vi "SMO Base Test Launcher.vi"() -> ()   [LabVIEW 2013]
uses:
  SMO.lvclass
  Typedefs/SMOState --Enum.ctl
panel:
  out "error out":errorcluster
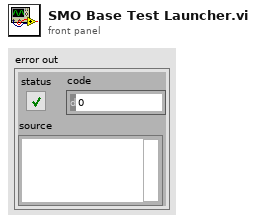
[diagram p1: front panel]
types:
  T1 = typedef "SMO.lvclass/Public Events.ctl" = cluster{"Error":refnum<user-event>, "State":refnum<user-event>, "Reserve State":refnum<user-event>}
  T2 = cluster{"Event Registration Refnum":refnum<event-registration>}
  T3 = typedef "SMO.lvclass/SMOState --Enum.ctl" = enum16{"unknown", "Created", "Started", "Stopped"}
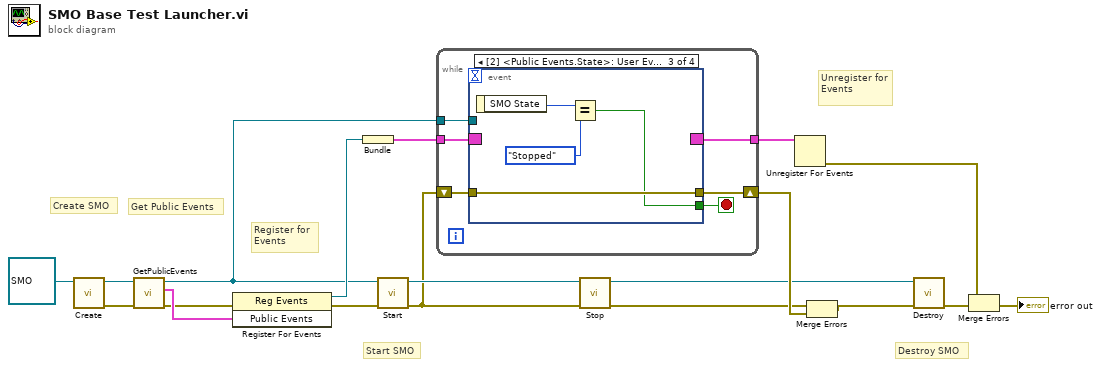
[diagram p0: block diagram]
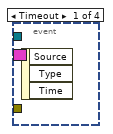
[diagram p2: hidden frame]
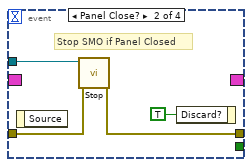
[diagram p3: hidden frame]
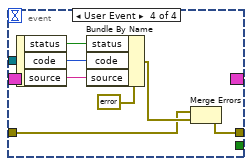
[diagram p4: hidden frame]
diagram:
  # "Get Public Events"
  # "Start SMO"
  # "Destroy SMO"
  # "Create SMO"
  # "Unregister for Events"
  # "Register for Events"
  n1 = call "Create.vi"("SMO"=refnum<class "SMO.lvclass"> refnum) -> ("error out"=w11:errorcluster, "SMO out"=w10:refnum<class "SMO.lvclass">)  [unwired: 8 in, 1 out]
  n2 = call "GetPublicEvents.vi"("error in (no error)"=w11, "SMO"=w10) -> ("error out"=w7:errorcluster, "Public Events"=w9:T1, "SMO out"=w8:refnum<class "SMO.lvclass">)  [unwired: 7 in]
  n3 = register-events(error in=w7, w9) -> (reference out=w13:refnum<event-registration>, error out=w12:errorcluster)  [unwired: 1 in]
  n4 = Bundle("Event Registration Refnum"=w13) -> (w18:T2)  [unwired: 1 in]
  n5 = call "Start.vi"("error in (no error)"=w12, "SMO"=w8) -> ("error out"=w2:errorcluster, "SMO out"=w4:refnum<class "SMO.lvclass">)  [unwired: 8 in]
  n6 = while {
    shift-right: [w24] -> w17
    shift-left: w2 -> [w23]
    tunnel: w18 -> [w22]
    tunnel: [w21] -> w19
    tunnel: w8 -> [w20]
    stop <- w25 stop-if-true
    n7 = event shown="[2] <Public Events.State>: User Event" {
      selector: w22 -> [_ _ _ _]
      dyn-events: [_ _ _ _] -> w21
      timeout: _ -> [_ _ _ _]
      tunnel: [_ _ w30 _] -> w25
      tunnel: w20 -> [_ w29 _ _]
      tunnel: [_ w28 w31 w34] -> w24
      tunnel: w23 -> [_ w27 w31 w35]
      event Timeout {
        n8 = event-data() -> ()  [unwired: 1 in, 3 out]
      }
      event Panel Close? {
        # "Stop SMO if Panel Closed"
        n9 = event-data() -> ()  [unwired: 1 in, 1 out]
        n10 = call "Stop.vi"("error in (no error)"=w27, "SMO"=w29) -> ("error out"=w28:errorcluster)  [unwired: 8 in, 1 out]
        n11 = event-data("Discard?"=TRUE ("OK")) -> ()  [unwired: 1 in, 1 out]
      }
      event User Event {
        n12 = event-data() -> ("SMO State"=w33:T3)  [unwired: 1 in]
        n13 = Equal?(x=w33, y=SMOState_--Enum."Stopped") -> (x = y?=w30:bool)
      }
      event User Event {
        n14 = event-data() -> ("status"=w40:bool, "code"=w39:i32, "source"=w38:string)  [unwired: 1 in]
        n15 = Bundle By Name(cluster=errorcluster {"status"=FALSE, "code"=0, "source"=""} ("error out"), "status"=w40, "code"=w39, "source"=w38) -> (w36:errorcluster)
        n16 = Merge Errors(w35, w36) -> (w34:errorcluster)
      }
    }
  }
  n17 = call "Stop.vi"("error in (no error)"=w2, "SMO"=w4) -> ("error out"=w1:errorcluster, "SMO out"=w3:refnum<class "SMO.lvclass">)  [unwired: 8 in]
  n18 = Unregister For Events(event registration refnum=w19) -> (error out=w16:errorcluster)  [unwired: 1 in]
  n19 = Merge Errors(w1, w17) -> (w6:errorcluster)
  n20 = call "Destroy.vi"("error in (no error)"=w6, "SMO"=w3) -> ("error out"=w14:errorcluster)  [unwired: 9 in]
  n21 = Merge Errors(w16, w14) -> (→"error out":errorcluster)
